vi "Update Version.vi"(8 "error in (no error)":errorcluster, 9 "Valid":bool, 10 "Library Version":T1, 11 "NI_AB_API_PPL in":refnum<class "NI_AB_API_PPL.lvclass">) -> (0 "error out":errorcluster, 2 "Updated":bool, 3 "NI_AB_API_PPL out":refnum<class "NI_AB_API_PPL.lvclass">)   [LabVIEW 2021, in "CIF Build Actions.lvlib"]
uses:
  CIF Build Actions.lvlib
  <vilib>/AppBuilder/AB_API/PPL/NI_AB_API_PPL.lvclass
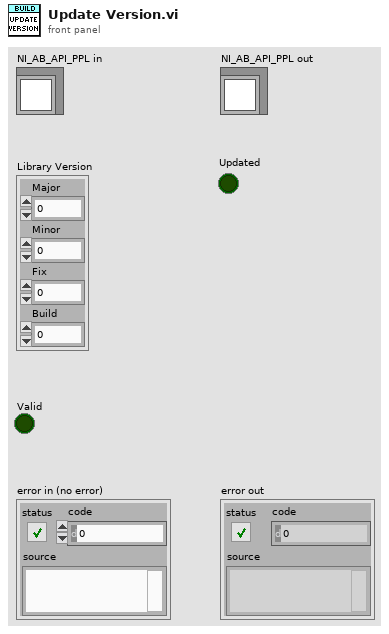
[diagram p1: front panel]
types:
  T1 = cluster{"Major":u16, "Minor":u16, "Fix":u16, "Build":u16}
  T2 = typedef "AB_API Version Number.ctl" = cluster{"Major":u16, "Minor":u16, "Fix":u16, "Build":u16}
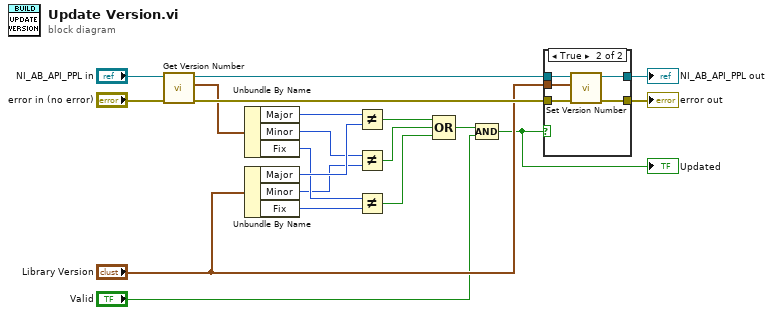
[diagram p0: block diagram]
diagram:
  n1 = call-dynamic "Get Version Number.vi"("error in (no error)"="error in (no error)", "NI_AB_API_Build in"="NI_AB_API_PPL in") -> ("error out"=w20:errorcluster, "Version number"=w14:T2, "NI_AB_API_Build out"=w19:refnum<class "NI_AB_API_PPL.lvclass">)  [unwired: 7 in]
  n2 = Unbundle By Name(w14) -> ("Major"=w12:u16, "Minor"=w8:u16, "Fix"=w9:u16)
  n3 = Unbundle By Name("Library Version") -> ("Major"=w11:u16, "Minor"=w7:u16, "Fix"=w10:u16)
  n4 = Not Equal?(x=w12, y=w11) -> (x != y?=w6:bool)
  n5 = Not Equal?(x=w8, y=w7) -> (x != y?=w5:bool)
  n6 = Not Equal?(x=w9, y=w10) -> (x != y?=w4:bool)
  n7 = Compound Arithmetic op=OR(w6, w5, w4) -> (w3:bool)
  n8 = Compound Arithmetic op=AND(w3, "Valid") -> (w1:bool)
  "Updated" <- w1
  n9 = case shown="True" w1 {
    tunnel: "Library Version" -> [_ w27]
    tunnel: w19 -> [w22 w26]
    tunnel: w20 -> [w21 w25]
    tunnel: [w22 w24] -> w15
    tunnel: [w21 w23] -> w16
    frame False {
    }
    frame True {
      n10 = call-dynamic "Set Version Number.vi"("error in (no error)"=w25, "Version number"=w27, "PPL in"=w26) -> ("error out"=w23:errorcluster, "PPL out"=w24:refnum<class "NI_AB_API_PPL.lvclass">)  [unwired: 7 in]
    }
  }
  "error out" <- w16
  "NI_AB_API_PPL out" <- w15
